vi "PH_HamamatsuCamera.configure ROI.vi"(0 "VI in":refnum<vi>, 1 "Cam Handle in":i32, 4 "Cam Error in":errorcluster, 5 "error in (no error)":errorcluster) -> (14 "VI out":refnum<vi>, 15 "Cam Handle out":i32, 18 "Cam Error out":errorcluster, 19 "error out":errorcluster)   [LabVIEW 2014, in "PH_HamamatsuCamera.lvlib"]
uses:
  PH_HamamatsuCamera.lvlib
  PH_HamamatsuCamera.ROI.ctl
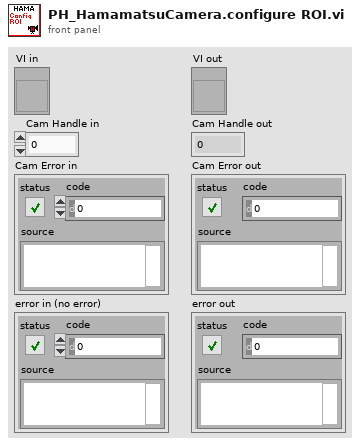
[diagram p1: front panel]
types:
  T1 = typedef "PH_HamamatsuCamera.lvlib/PH_HamamatsuCamera.i attribute.ctl" = cluster{"Gui Refs":cluster{"Camera Details":refnum<vi>, "ROI":refnum<vi>, "Set ROI to Maximum":refnum<vi>, "Trigger Parameters":refnum<vi>, "Brightness":refnum<vi>, "Shutter":refnum<vi>, "Gain":refnum<vi>, "Trigger Timeout":refnum<vi>, "Trigger Polarity":refnum<vi>, "Trigger Mode":refnum<vi>, "Parameters":refnum<vi>, "Set Cam Parameter":refnum<vi>, "Parameter to set":refnum<vi>, "Value to set":refnum<vi>}, "Cam":cluster{"Handle":i32, "Details":cluster{"Model":string, "Camera ID":string, "Firmware":string}, "Buffer Info":cluster{"height":u32, "width":u32, "datatype":u32}}, "H Offset":cluster{"Value":i32, "Minimum":i32, "Maximum":i32, "Increment":i32}, "V Offset":cluster{"Value":i32, "Minimum":i32, "Maximum":i32, "Increment":i32}, "H Width":cluster{"Value":i32, "Minimum":i32, "Maximum":i32, "Increment":i32}, "V Width":cluster{"Value":i32, "Minimum":i32, "Maximum":i32, "Increment":i32}, "Trigger Parameters":T2, "Trigger Timeout":u32, "Parameters":T3[], "Indicees Cam Parameters":cluster{"Brightness":i32, "Shutter":i32, "Gain":i32}, "Wanted Values":cluster{"Trigger Settings":T2[], "ROI":T4[], "Parameter":cluster{"Name":string, "Value":dbl}[]}}
  T2 = typedef "PH_HamamatsuCamera.lvlib/PH_HamamatsuCamera.Trigger Parameter.ctl" = cluster{"Mode":u32, "Polarity":u32, "Times":u32, "Delay":dbl}
  T3 = typedef "PH_HamamatsuCamera.lvlib/PH_HamamatsuCamera.Parameter Set.ctl" = cluster{"Parameter":string, "Value":dbl, "Writable":bool, "Range":cluster{"min":dbl, "max":dbl, "step":dbl}, "Default":dbl, "Value Names":cluster{"Name":string, "Value":dbl}[], "Text Values":bool}
  T4 = typedef "PH_HamamatsuCamera.lvlib/PH_HamamatsuCamera.ROI.ctl" = cluster{"Horizontal Offset":i32, "Vertical Offset":i32, "Horizontal Width":i32, "Vertical Width":i32}
  T5 = cluster{"Horizontal Offset":i32, "Vertical Offset":i32, "Horizontal Width":i32, "Vertical Width":i32}
  T6 = cluster{"Value":i32, "Minimum":i32, "Maximum":i32, "Increment":i32}
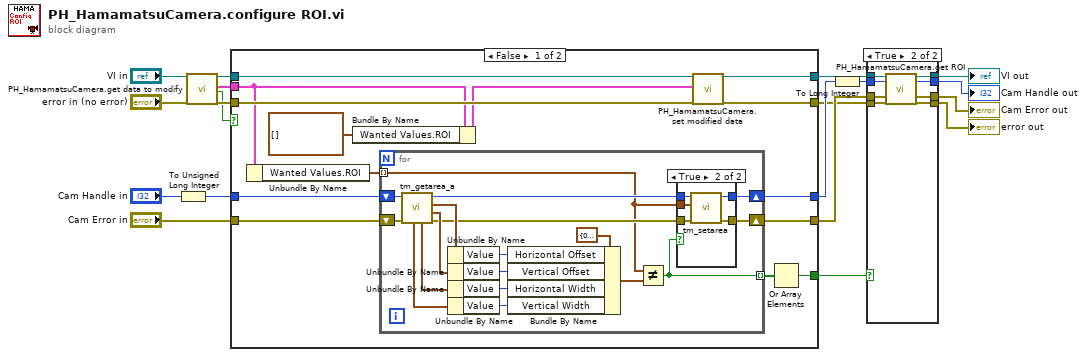
[diagram p0: block diagram]
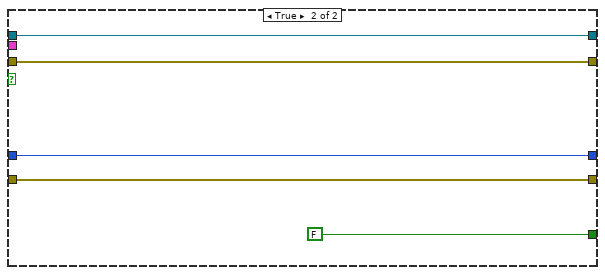
[diagram p3: hidden frame]
diagram:
  n1 = To Unsigned Long Integer(number="Cam Handle in") -> (unsigned 32bit integer=w1:u32)
  n2 = call "PH_HamamatsuCamera.get data to modify.vi"("i ref in"="VI in", "error in (no error)"="error in (no error)") -> ("i ref out"=w5:refnum<vi>, "i attribute"=w6:T1, "timed out"=w2:bool, "error out"=w9:errorcluster)  [unwired: 14 in]
  n3 = case shown="False" w2 {
    tunnel: [w33 w61] -> w16
    tunnel: [w32 w60] -> w15
    tunnel: "Cam Error in" -> [w31 w60]
    tunnel: [w20 FALSE] -> w12
    tunnel: w1 -> [w29 w61]
    tunnel: w9 -> [w28 w62]
    tunnel: [w27 w62] -> w7
    tunnel: w6 -> [w26 _]
    tunnel: w5 -> [w25 w63]
    tunnel: [w24 w63] -> w4
    frame False {
      n4 = Unbundle By Name(w26) -> ("Wanted Values.ROI"=w21:T4[])
      n5 = Bundle By Name(cluster=w26, "Wanted Values.ROI"=T4[] []) -> (w23:T1)
      n6 = for {
        tunnel: [w48] -> w30 mode=indexing
        tunnel: w21 -> [w34] mode=indexing
        shift-right: [w50] -> w32
        shift-left: w31 -> [w49]
        shift-right: [w51] -> w33
        shift-left: w29 -> [w37]
        n7 = call <userlib>:"tm_getarea_a.vi"("error in (no error)"=w49, "Handle in"=w37) -> ("error out"=w38:errorcluster, "V Offset"=w40:T6, "H Offset"=w39:T6, "Handle out"=w36:u32, "H Width"=w41:T6, "V Width"=w42:T6)  [unwired: 4 in]
        n8 = Unbundle By Name(w39) -> ("Value"=w43:i32)
        n9 = Unbundle By Name(w40) -> ("Value"=w44:i32)
        n10 = Unbundle By Name(w41) -> ("Value"=w45:i32)
        n11 = Unbundle By Name(w42) -> ("Value"=w46:i32)
        n12 = Bundle By Name(cluster=T5 {"Horizontal Offset"=0, "Vertical Offset"=0, "Horizontal Width"=0, "Vertical Width"=0} ("Sub Region"), "Horizontal Offset"=w43, "Vertical Offset"=w44, "Horizontal Width"=w45, "Vertical Width"=w46) -> (w35:T5)
        n13 = Not Equal?(x=w34, y=w35) -> (x != y?=w48:bool)
        n14 = case shown="True" w48 {
          tunnel: w36 -> [w52 w58]
          tunnel: w38 -> [w53 w57]
          tunnel: w34 -> [_ w56]
          tunnel: [w53 w55] -> w50
          tunnel: [w52 w54] -> w51
          frame False {
          }
          frame True {
            n15 = call <userlib>:"tm_setarea.vi"("error in (no error)"=w57, "Sub Region"=w56, "Handle in"=w58) -> ("error out"=w55:errorcluster, "Handle out"=w54:u32)  [unwired: 7 in]
          }
        }
      }
      n16 = call "PH_HamamatsuCamera.set modified data.vi"("i ref in"=w25, "i attribute"=w23, "error in (no error)"=w28) -> ("i ref out"=w24:refnum<vi>, "error out"=w27:errorcluster)  [unwired: 15 in]
      n17 = Or Array Elements(Boolean array=w30) -> (logical OR=w20:bool)
    }
    frame True {
    }
  }
  n18 = To Long Integer(number=w16) -> (32bit integer=w19:i32)
  n19 = case shown="True" w12 {
    tunnel: [w66 w75] -> w3
    tunnel: [w67 w74] -> w11
    tunnel: w4 -> [w67 w73]
    tunnel: w7 -> [w66 w72]
    tunnel: w15 -> [w64 w71]
    tunnel: w19 -> [w65 w70]
    tunnel: [w65 w69] -> w17
    tunnel: [w64 w68] -> w18
    frame False {
    }
    frame True {
      n20 = call "PH_HamamatsuCamera.get ROI.vi"("i ref in"=w73, "Cam Handle in"=w70, "Cam Error in"=w71, "error in (no error)"=w72) -> ("i ref out"=w74:refnum<vi>, "Handle out"=w69:i32, "Cam Error out"=w68:errorcluster, "error out"=w75:errorcluster)  [unwired: 12 in]
    }
  }
  "Cam Error out" <- w18
  "Cam Handle out" <- w17
  "VI out" <- w11
  "error out" <- w3
